vi "Set DO State (automation mode) Multiple.vi"(8 "error in (no error)":errorcluster, 9 "Values":bool[](array[boolean]), 10 "DOs":T1[](array[typedef]), 11 "DAQ in":refnum<class "DAQ.lvclass">) -> (0 "error out":errorcluster, 3 "DAQ out":refnum<class "DAQ.lvclass">)   [LabVIEW 2022 SP3, in "DAQ.lvclass"]
uses:
  DAQ.lvclass
  DAQ.lvclass/DAQ.ctl
  IO/Typedefs/ICP2-DO Channel Names.ctl
  IO/IO.lvclass
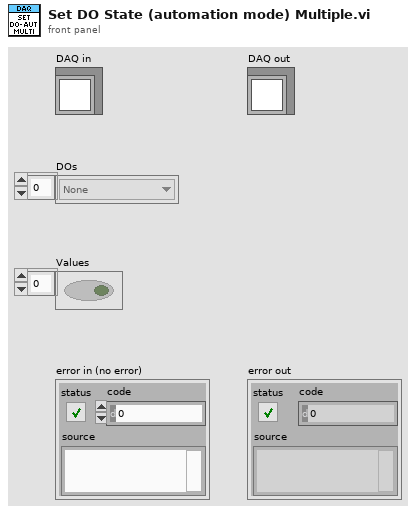
[diagram p1: front panel]
types:
  T1 = typedef "IO.lvclass/ICP2-DO Channel Names.ctl" = enum16{"None", "Meniscus Valve Open - R1", "Meniscus Valve Open - R2", "Meniscus Valve Open - R3", "Meniscus Valve Open - R4", "Meniscus Valve Open - R5", "Meniscus Valve Open - R6", "Ink Flow Valve Open - R1", "Ink Flow Valve Open - R2", "Ink Flow Valve Open - R3", "Ink Flow Valve Open - R4", "Ink Flow Valve Open - R5", "Ink Flow Valve Open - R6", "SW_LED - Ink Valve - R1", "SW_LED - Ink Valve - R2", "SW_LED - Ink Valve - R3", "Recirc Pump On - R1", "Recirc Pump On - R2", "Recirc Pump On - R3", "Recirc Pump On - R4", "Recirc Pump On - R5", "Recirc Pump On - R6", "SW_LED - Ink Valve - R4", "SW_LED - Ink Valve - R5", "SW_LED - Ink Valve - R6"}
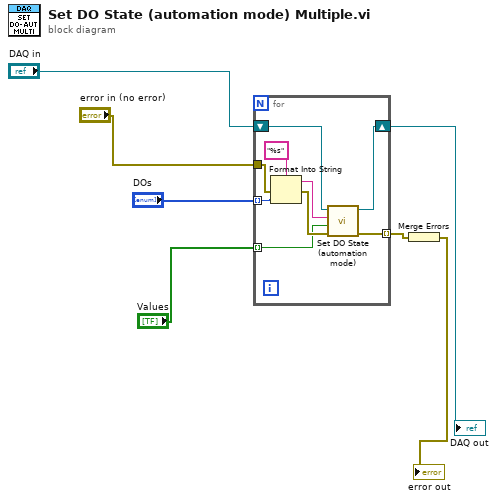
[diagram p0: block diagram]
diagram:
  n1 = for {
    tunnel: "DOs" -> [w13] mode=indexing
    shift-right: [w11] -> w4
    shift-left: "DAQ in" -> [w12]
    tunnel: [w10] -> w5 mode=indexing
    tunnel: "Values" -> [w9] mode=indexing
    tunnel: "error in (no error)" -> [w8]
    n2 = Format Into String(format string="%s", error in=w8, w13) -> (resulting string=w15:string, error out=w16:errorcluster)  [unwired: 1 in]
    n3 = call "Set DO State (automation mode).vi"("error in (no error)"=w16, "State"=w9, "DO IOName"=w15, "DAQ"=w12) -> ("error out"=w10:errorcluster, "DAQ"=w11:refnum<class "DAQ.lvclass">)  [unwired: 6 in]
  }
  "DAQ out" <- w4
  n4 = Merge Errors(w5) -> (→"error out":errorcluster)
